vi "Mathematica.global.vi"() -> ()   [LabVIEW 2014]
uses:
  D:/Desktop/app/LabVIEW/Wolfram.NETLink.dll
  Wolfram.NETLink.dll
panel:
  out "Mathematica":refnum<k24>
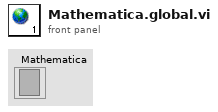
[diagram p1: front panel]
diagram:
